vi "SwissSPAD Live_Get SS3 FPGA Parameters.vi"(6 "Live Mode":bool, 8 "Error In":errorcluster, 10 "Bifile Path":path, 11 "SS3 DAQ Parameters":T1 {"Gate Width (ns)" min=0.0 max=100.0 format="%#_5g"; "# Sets" min=1}) -> (0 "Error Out":errorcluster, 1 "# 8-bit Images per Set":u32, 2 "SS3 FPGA DAQ Parameters":u32[](array[numeric]), 3 "SS3 FPGA DAQ Addresses":i32[](array[numeric]) format="%x", 5 "Discard First Image":bool)   [LabVIEW 2021]
uses:
  SwissSPAD Live_SS3 DAQ Parameters.ctl
  SwissSPAD Live_SS3 Gate Definition.ctl
  SS3 Gate Width Definition Mode.ctl
  <vilib>/Utility/error.llb/Error Cluster From Error Code.vi
  <vilib>/ErrorRing/Error Ring.xnode
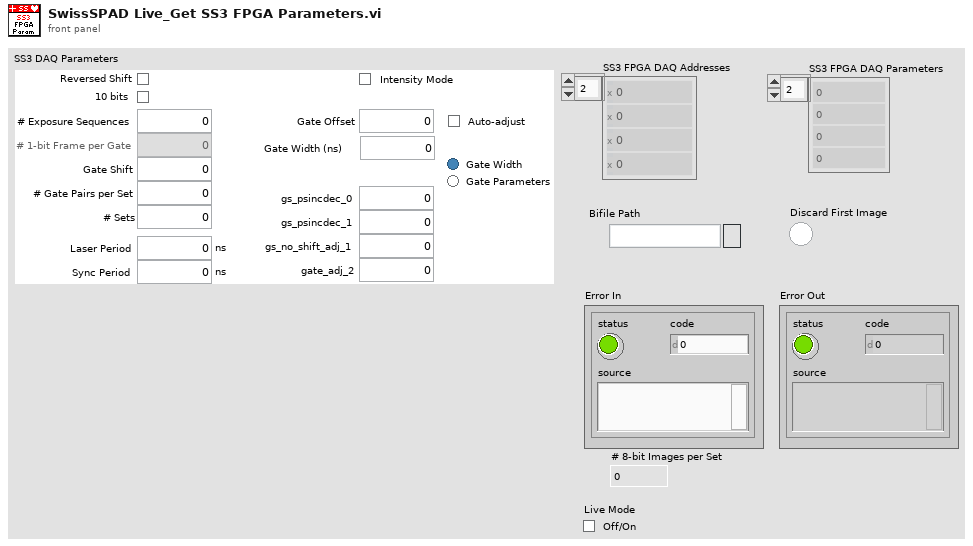
[diagram p1: front panel]
types:
  T1 = typedef "SwissSPAD Live_SS3 DAQ Parameters.ctl" = cluster{"10 bits":bool, "# Exposure Sequences":u32, "# 1-bit Frame per Gate":u32, "Gate Shift":u32, "# Gate Pairs per Set":u32, "# Sets":u32, "Laser Period":dbl[unit], "Sync Period":dbl[unit], "Gate Offset":u32, "Auto-adjust Gate Offset":bool, "Gate Definition":T2, "Gate Width (ns)":dbl, "Reversed Shift":bool, "Intensity Mode":bool, "Gate Definition Mode":T3}
  T2 = typedef "SwissSPAD Live_SS3 Gate Definition.ctl" = cluster{"gs_psincdec_0":u32, "gs_psincdec_1":u32, "gs_no_shift_adj_1":u32, "gate_adj_2":u32}
  T3 = typedef "SS3 Gate Width Definition Mode.ctl" = enum32{"Item 0", "Item 1"}
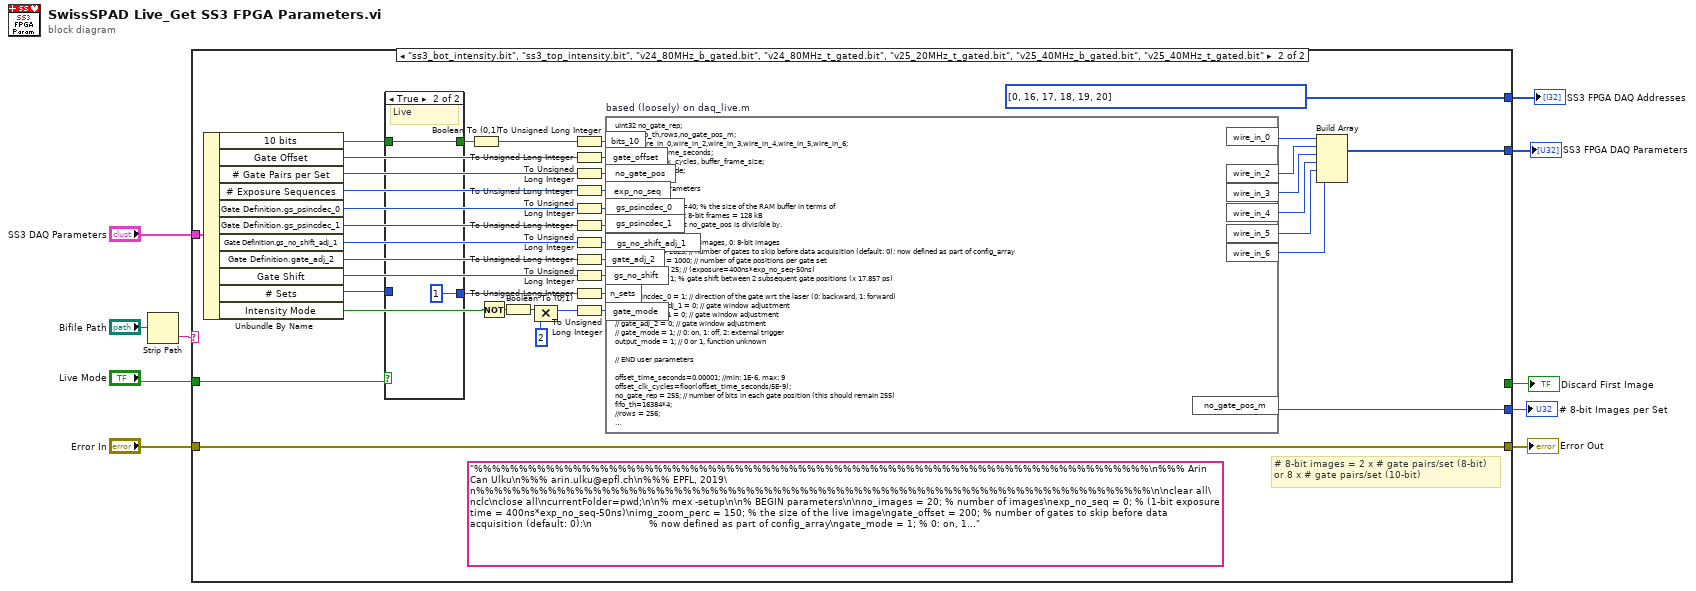
[diagram p0: block diagram]
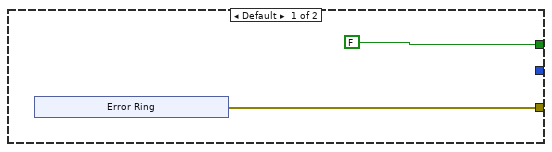
[diagram p2: hidden frame]
diagram:
  n1 = Strip Path(path="Bifile Path") -> (name=w5:string)  [unwired: 1 out]
  n2 = case shown="\"ss3_bot_intensity.bit\", \"ss3_top_intensity.bit\", \"v24_80MHz_b_gated.bit\", \"v24_80MHz_t_gated.bit\", \"v25_20MHz_t_gated.bit\", \"v25_40MHz_b_gated.bit\", \"v25_40MHz_t_gated.bit\"" w5 {
    tunnel: [_ w54] -> w10
    tunnel: [_ i32[] [0, 16, 17, 18, 19, 20] ("SS2 FPGA DAQ Addresses")] -> w9
    tunnel: "SS3 DAQ Parameters" -> [_ w52]
    tunnel: [_ w44] -> w8
    tunnel: "Live Mode" -> [_ w39]
    tunnel: "Error In" -> [_ w21]
    tunnel: [w12 w21] -> w4
    tunnel: [FALSE ("Discard First Image") _] -> w2
    frame Default {
      n3 = xnode "Error Ring"() -> ("error out"=w12:errorcluster)
    }
    frame "ss3_bot_intensity.bit", "ss3_top_intensity.bit", "v24_80MHz_b_gated.bit", "v24_80MHz_t_gated.bit", "v25_20MHz_t_gated.bit", "v25_40MHz_b_gated.bit", "v25_40MHz_t_gated.bit" {
      (unwired) "%%%%%%%%%%%%%%%%%%%%%%%%%%%%%%%%%%%%%%%%%%%%%%%%%%%%%%%%%%%%%%%%%%%%%%%%%%%\n%%% Arin Can Ulku\n%%% arin.ulku@epfl.ch\n%%% EPFL, 2019\n%%%%%%%%%%%%%%%%%%%%%%%%%%%%%%%%%%%%%%%%%%%%%%%%%%%%%%%%%%%%%%%%%%%%%%%%%%%\n\nclear all\nclc\nclose all\ncurrentFolder=pwd;\n\n% mex -setup\n\n% BEGIN parameters\n\nno_images = 20; % number of images\nexp_no_seq = 0; % (1-bit exposure time = 400ns*exp_no_seq-50ns)\nimg_zoom_perc = 150; % the size of the live image\ngate_offset = 200; % number of gates to skip before data acquisition (default: 0):\n                   % now defined as part of config_array\ngate_mode = 1; % 0: on, 1: off, 2: external trigger\noutput_mode = 0; % choose 0 or 1\n\ngs_psincdec_0 = 1; % direction of the gate wrt the laser (0: backward, 1: forward)\ngs_no_shift_adj_1 = 100; % gate window adjustment\ngs_psincdec_1 = 0; % gate window adjustment\n\n% END parameters\n\ngs_no_shift = 2;\noffset_time_seconds=0.001; %% min: 1E-6, max: 9\noffset_clk_cycles=floor(offset_time_seconds/(5E-9));\nfifo_th=20*256;\n\nsetenv('MW_MINGW32_LOC','C:\\TDM-GCC-32')\nloadlibrary('okFrontPanel', 'okFrontPanelDLL.h', 'notempdir');\ndev = openFPGA();\n\n% bitfile = [currentFolder '\\bit_file\\TOP.bit'];\n% bitfile = [currentFolder '\\bit_file\\TOP.bit'];\n%bitfile = [currentFolder '\\bit_file\\TOP_80_MHz_v2.bit'];\n% bitfile = [currentFolder '\\bit_file\\TOP_80_MHz.bit'];\nz_status=configureFPGA(dev, bitfile);\n\nwire_in_0=gs_psincdec_0+gs_psincdec_1*2^1+gs_no_shift_adj_1*2^4+gate_mode*2^20+output_mode*2^22;\nsetwireinvalue(dev,int32(hex2dec('00')),wire_in_0,wire_in_0)\nupdatewireins(dev)\nwire_in_2=no_images*2^8;\nsetwireinvalue(dev,int32(hex2dec('10')),wire_in_2,wire_in_2)\nupdatewireins(dev)\nwire_in_3=exp_no_seq+gate_offset*2^16;\nsetwireinvalue(dev,int32(hex2dec('11')),wire_in_3,wire_in_3)\nupdatewireins(dev)\nwire_in_4=gs_no_shift;\nsetwireinvalue(dev,int32(hex2dec('12')),wire_in_4,wire_in_4)\nupdatewireins(dev)\nwire_in_5=fifo_th;\nsetwireinvalue(dev,int32(hex2dec('13')),wire_in_5,wire_in_5)\nupdatewireins(dev)\nwire_in_6=offset_clk_cycles;\nsetwireinvalue(dev,int32(hex2dec('14')),wire_in_6,wire_in_6)\nupdatewireins(dev)\n\nA=zeros(256,512,'uint8');\n\nfor i=1:no_images\n    \n    activatetriggerin(dev,int32(hex2dec('40')),0)\n    activatetriggerin(dev,int32(hex2dec('40')),1)\n\n    D=readfromblockpipeout(dev,int32(hex2dec('A0')),(16*256*4),(512*256));\n    for row = 1:256\n        for col = 1:512\n            temp=floor((col-1)/128);\n            col1=4*(col-temp*128)-3+temp;\n            A(row,col1) = D((row-1)*512+col);\n        end\n    end\n    B=A(7:255,1:500);\n    mn=mean(B(:))\n    imshow(A, 'InitialMagnification', img_zoom_perc);\n%     imwrite(A,[currentFolder '\\image.tiff'],'Compression','none');\nend\n\ncloseFPGA(dev);\n\ndisp('DONE.')\nbeep\n"
      # "# 8-bit images = 2 x # gate pairs/set (8-bit)\nor 8 x # gate pairs/set (10-bit)"
      n4 = Unbundle By Name(w52) -> ("10 bits"=w38:bool, "Gate Offset"=w34:u32, "# Gate Pairs per Set"=w50:u32, "# Exposure Sequences"=w49:u32, "Gate Definition.gs_psincdec_0"=w43:u32, "Gate Definition.gs_psincdec_1"=w42:u32, "Gate Definition.gs_no_shift_adj_1"=w41:u32, "Gate Definition.gate_adj_2"=w40:u32, "Gate Shift"=w48:u32, "# Sets"=w36:u32, "Intensity Mode"=w20:bool)
      n5 = case shown="True" w39 {
        tunnel: w38 -> [w59 w60]
        tunnel: [w59 w60] -> w37
        tunnel: w36 -> [w58 _]
        tunnel: [w58 u32 1 ("# Sets")] -> w35
        frame False {
          # "Recording"
        }
        frame True {
          # "Live"
        }
      }
      n6 = Boolean To (0,1)(Boolean=w37) -> (0, 1=w51:i16)
      n7 = Not(x=w20) -> (.not. x?=w17:bool)
      n8 = Boolean To (0,1)(Boolean=w17) -> (0, 1=w19:i16)
      n9 = Compound Arithmetic op=MULTIPLY(w19, i16 2 ("value")) -> (w22:i16)
      n10 = To Unsigned Long Integer(number=w51) -> (unsigned 32bit integer=w33:u32)
      n11 = To Unsigned Long Integer(number=w34) -> (unsigned 32bit integer=w32:u32)
      n12 = To Unsigned Long Integer(number=w50) -> (unsigned 32bit integer=w24:u32)
      n13 = To Unsigned Long Integer(number=w49) -> (unsigned 32bit integer=w25:u32)
      n14 = To Unsigned Long Integer(number=w43) -> (unsigned 32bit integer=w27:u32)
      n15 = To Unsigned Long Integer(number=w42) -> (unsigned 32bit integer=w28:u32)
      n16 = To Unsigned Long Integer(number=w41) -> (unsigned 32bit integer=w29:u32)
      n17 = To Unsigned Long Integer(number=w40) -> (unsigned 32bit integer=w30:u32)
      n18 = To Unsigned Long Integer(number=w48) -> (unsigned 32bit integer=w26:u32)
      n19 = To Unsigned Long Integer(number=w35) -> (unsigned 32bit integer=w31:u32)
      n20 = To Unsigned Long Integer(number=w22) -> (unsigned 32bit integer=w23:u32)
      n21 = formula code="uInt32 no_gate_rep;\nuInt32 fifo_th,rows,no_gate_pos_m;\nuInt32 wire_in_0,wire_in_2,wire_in_3,wire_in_4,wire_in_5,wire_in_6;\nfloat64 offset_time_seconds;\nuInt32 offset_clk_cycles, buffer_frame_size;\nuInt32 output_mode;\n\n// BEGIN user parameters\n\n// buffer_frame_size=40; % the size of the RAM buffer in terms of \n// equivalent 256*512 8-bit frames = 128 kB\n// choose a value that no_gate_pos is divisible by.\n\n// bits_10 = 0; // 1: 10-bit images, 0: 8-bit images\n// gate_offset = 2025; // number of gates to skip before data acquisition (default: 0): now defined as part of config_array\n// no_gate_pos = 1000; // number of gate positions per gate set\n// exp_no_seq = 25; // (exposure=400ns*exp_no_seq-50ns)\n// gs_no_shift = 1; % gate shift between 2 subsequent gate positions (x 17.857 ps)\n\n// gs_psincdec_0 = 1; // direction of the gate wrt the laser (0: backward, 1: forward)\n// gs_no_shift_adj_1 = 0; // gate window adjustment\n// gs_psincdec_1 = 0; // gate window adjustment\n// gate_adj_2 = 0; // gate window adjustment\n// gate_mode = 1; // 0: on, 1: off, 2: external trigger\noutput_mode = 1; // 0 or 1, function unknown\n\n// END user parameters\n\noffset_time_seconds=0.00001; //min: 1E-6, max: 9\noffset_clk_cycles=floor(offset_time_seconds/5E-9);\nno_gate_rep = 255; // number of bits in each gate position (this should remain 255)\nfifo_th=16384*4;\n//rows = 256;\n\nno_gate_pos_m = (bits_10 ==1) ? no_gate_pos*8 : no_gate_pos*2;\n//buffer_frame_size = (bits_10 ==1) ? 8 : 2;\n//= no_gate_pos_m; // e.g. bits_10 = 1, no_gate_pos = 100 >> buffer = 50 MB\n//no_gate_pos_m *= n_sets; \n\n//no_rows = rows-1;\n//frames=no_gate_rep;\n\nwire_in_0=gs_psincdec_0+gs_psincdec_1*2**1+gs_no_shift_adj_1*2**4 +\n    bits_10*2**19 + gate_mode*2**20 + output_mode*2**22 + gate_adj_2*2**23 ;\nwire_in_2=no_gate_pos_m*2**8;\nwire_in_3=exp_no_seq+gate_offset*2**16;\nwire_in_4=gs_no_shift;\nwire_in_5=fifo_th;\nwire_in_6=offset_clk_cycles;" "based (loosely) on daq_live.m"("bits_10"=w33, "gate_offset"=w32, "no_gate_pos"=w24, "exp_no_seq"=w25, "gs_psincdec_0"=w27, "gs_psincdec_1"=w28, "gs_no_shift_adj_1"=w29, "gate_adj_2"=w30, "gs_no_shift"=w26, "n_sets"=w31, "gate_mode"=w23) -> ("wire_in_0"=w57:u32, "wire_in_2"=w56:u32, "wire_in_3"=w55:u32, "no_gate_pos_m"=w44:u32, "wire_in_4"=w47:u32, "wire_in_5"=w46:u32, "wire_in_6"=w45:u32)
      n22 = Build Array(w57, w56, w55, w47, w46, w45) -> (w54:u32[])
    }
  }
  "SS3 FPGA DAQ Parameters" <- w10
  "Error Out" <- w4
  "SS3 FPGA DAQ Addresses" <- w9
  "# 8-bit Images per Set" <- w8
  "Discard First Image" <- w2
